vi "Initialization VI.vi"(8 "error in (no error)":errorcluster, 10 "Custom XML":string, 11 "Device Item Ref in":T1 format="%.0x") -> (0 "error out":errorcluster, 3 "Device Item Ref out":T1 format="%.0x")   [LabVIEW 2019, in "Instrument Addon System Explorer.lvlib"]
uses:
  Instrument Addon System Explorer.lvlib
  <vilib>/NI VeriStand/Custom Device API/Custom Device Item Ref.ctl
  Addon Shared/Types/FG Control.ctl
  Addon Shared/Constants.vi
  <vilib>/NI VeriStand/Custom Device API/NI VeriStand - Get Item Property.vi
  <vilib>/NI VeriStand/Custom Device API/Get Item Property (String).vi
  <vilib>/NI VeriStand/Custom Device API/NI VeriStand - Set Item Property.vi
  <vilib>/NI VeriStand/Custom Device API/Set Item Property (String).vi
  Addon Shared/Instrument Addon Shared.lvlib
  <vilib>/NI VeriStand/Custom Device API/Custom Device API.lvlib
  <vilib>/NI/NI VeriStand Custom Device Import and Export Tool/ImportExport.lvlib
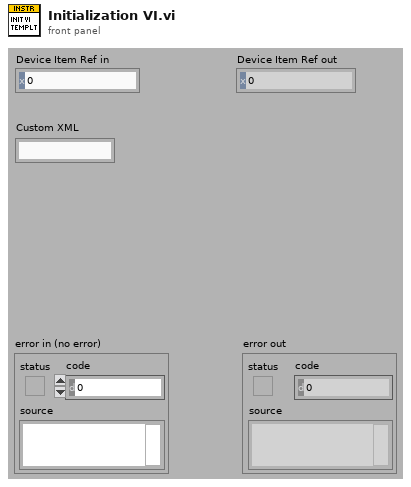
[diagram p1: front panel]
types:
  T1 = typedef "Custom Device API.lvlib/Custom Device Item Ref.ctl" = u64
  T2 = typedef "Instrument Addon Shared.lvlib/FG Control.ctl" = enum16{"Get", "Set"}
  T3 = typedef "Instrument Addon System Explorer.lvlib/Initial User Selection.ctl" = cluster{"Protocol":string}
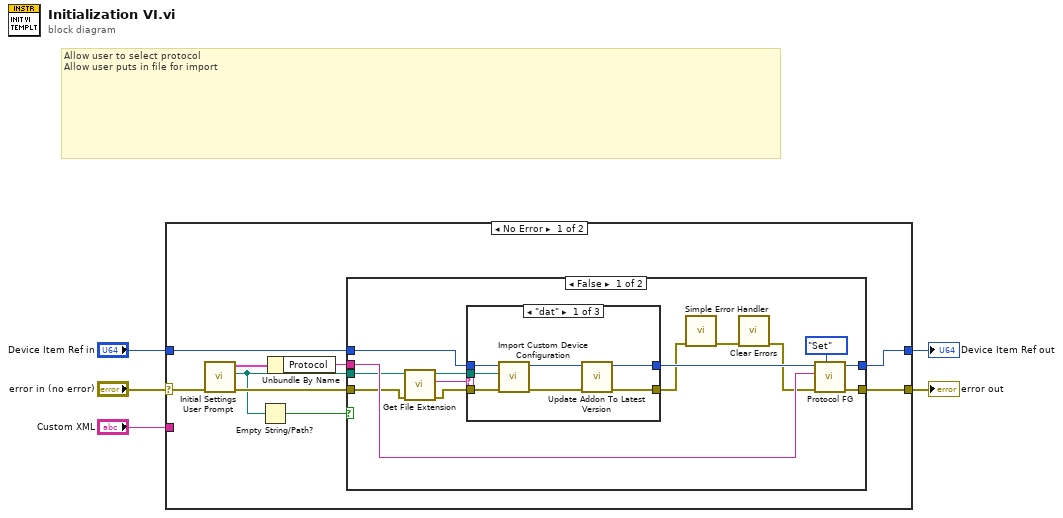
[diagram p0: block diagram]
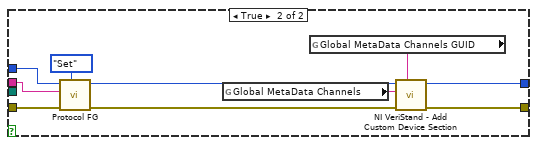
[diagram p4: hidden frame]
diagram:
  # "Allow user to select protocol\nAllow user puts in file for import"
  n1 = case shown="No Error" "error in (no error)" {
    selector: "error in (no error)" -> [w14 w50]
    tunnel: [w12 w50] -> w5
    tunnel: [w8 w49] -> w3
    tunnel: "Device Item Ref in" -> [w9 w49]
    tunnel: "Custom XML" -> [_ _]
    frame No Error {
      n2 = call "Initial Settings User Prompt.vi"("error in (no error)"=w14) -> ("error out"=w13:errorcluster, "Path out"=w6:path, "Initial Settings"=w11:T3)  [unwired: 8 in]
      n3 = Empty String/Path?(string/path=w6) -> (empty?=w7:bool)
      n4 = Unbundle By Name(w11) -> ("Protocol"=w10:string)
      n5 = case shown="False" w7 {
        tunnel: w13 -> [w17 w48]
        tunnel: [w26 w41] -> w12
        tunnel: w10 -> [w23 w42]
        tunnel: w9 -> [w28 w47]
        tunnel: [w24 w40] -> w8
        tunnel: w6 -> [w19 _]
        frame False {
          n6 = call <vilib>:"Get File Extension.vi"("error in (no error)"=w17, "file"=w19) -> ("error out"=w16:errorcluster, "lowercase file extension"=w15:string, "dup file"=w18:path)  [unwired: 5 in, 2 out]
          n7 = case shown="\"dat\"" w15 {
            tunnel: w16 -> [w35 w37 w38]
            tunnel: w28 -> [w34 w36 w39]
            tunnel: w18 -> [w33 _ _]
            tunnel: [w29 w36 w39] -> w25
            tunnel: [w31 w37 w38] -> w21
            frame "dat" {
              n8 = call <vilib>:"Import Custom Device Configuration.vi"("error in (no error)"=w35, "Path"=w33, "NodeID"=w34) -> ("error out"=w32:errorcluster, "NodeID out"=w30:u64)  [unwired: 6 in, 1 out]
              n9 = call "Update Addon To Latest Version.vi"("error in (no error)"=w32, "Device Item Ref in"=w30) -> ("error out"=w31:errorcluster, "Device Item Ref out"=w29:T1)  [unwired: 8 in]
            }
            frame "xml" {
            }
            frame Default {
            }
          }
          n10 = call <vilib>:"Simple Error Handler.vi"("error in (no error)"=w21) -> ("error out"=w22:errorcluster)  [unwired: 4 in, 4 out]
          n11 = call <vilib>:"Clear Errors.vi"("error in (no error)"=w22) -> ("error out"=w20:errorcluster)  [unwired: 5 in, 1 out]
          n12 = call "Protocol FG.vi"("Action"=FG_Control."Set", "error in (no error)"=w20, "Protocol"=w23, "Device Item Ref in"=w25) -> ("error out"=w26:errorcluster, "Item Ref out"=w24:T1)  [unwired: 5 in, 1 out]
        }
        frame True {
          n13 = call "Protocol FG.vi"("Action"=FG_Control."Set", "error in (no error)"=w48, "Protocol"=w42, "Device Item Ref in"=w47) -> ("error out"=w41:errorcluster, "Item Ref out"=w46:T1)  [unwired: 5 in, 1 out]
          n14 = global read "Constants.vi" "Global MetaData Channels"() -> (w43:string)
          n15 = global read "Constants.vi" "Global MetaData Channels GUID"() -> (w44:string)
          n16 = call <vilib>:"NI VeriStand - Add Custom Device Section.vi"("GUID (Default Section)"=w44, "Section Name"=w43, "Parent Ref in"=w46) -> ("Parent Ref out"=w40:T1)  [unwired: 5 in, 3 out]
        }
      }
    }
    frame Error {
    }
  }
  "error out" <- w5
  "Device Item Ref out" <- w3
